vi "ReadReply.vi"(6 "length":i32=-1, 8 "error in (no error)":errorcluster, 9 "Type":enum16{"Header", "Body"}(ring)=enum."Body", 10 "timeout ms (60000)":i32, 11 "TCP in":refnum<k5>) -> (0 "error out":errorcluster, 2 "String":string, 3 "TCP out":refnum<k5>)   [LabVIEW 2019]
panel:
  out "last line":string
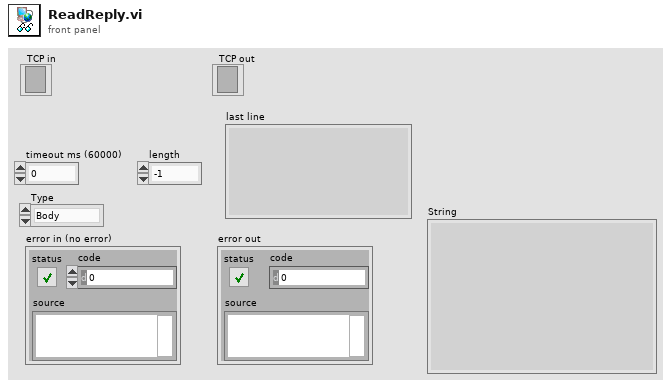
[diagram p1: front panel]
types:
  T1 = enum16{"Standard", "Buffered", "CRLF", "Immediate"}
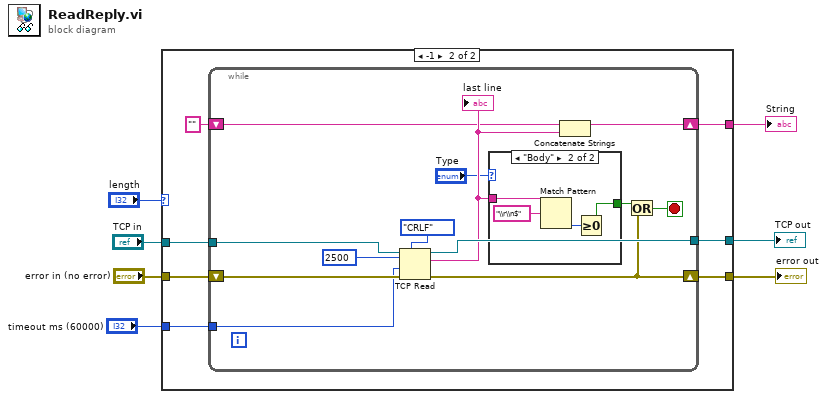
[diagram p0: block diagram]
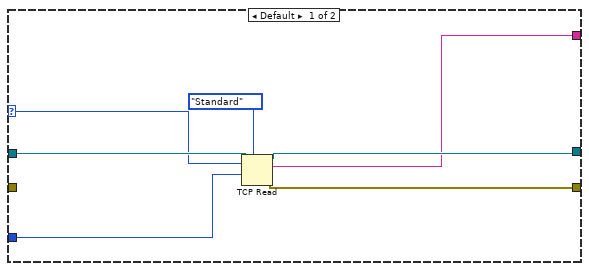
[diagram p2: hidden frame]
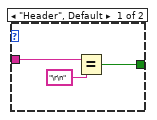
[diagram p3: hidden frame]
diagram:
  n1 = case shown="-1" "length" {
    selector: "length" -> [w11 _]
    tunnel: [w9 w21] -> w7
    tunnel: "error in (no error)" -> [_ w20]
    tunnel: "TCP in" -> [w13 w19]
    tunnel: [w10 w18] -> w4
    tunnel: [w8 w17] -> w3
    tunnel: "timeout ms (60000)" -> [w12 w15]
    frame Default {
      n2 = TCP Read(connection ID=w13, bytes to read=w11, 7:T1."Standard" ("mode (standard)"), 9:w12) -> (connection ID out=w10:refnum<k5>, data out=w8:string, error out=w9:errorcluster)  [unwired: 1 in]
    }
    frame -1 {
      n3 = while {
        shift-right: [w28] -> w21
        shift-left: w20 -> [w34]
        tunnel: w19 -> [w33]
        tunnel: [w32] -> w18
        shift-right: [w31] -> w17
        shift-left: "" ("data out") -> [w26]
        tunnel: w15 -> [w22]
        stop <- w29 stop-if-true
        n4 = TCP Read(connection ID=w33, bytes to read=2500, error in (no error)=w34, 7:T1."CRLF" ("mode (standard)"), 9:w22) -> (connection ID out=w32:refnum<k5>, data out=w27:string, error out=w28:errorcluster)
        "last line" <- w27
        n5 = case shown="\"Body\"" "Type" {
          tunnel: [w36 w38] -> w30
          tunnel: w27 -> [w35 w40]
          frame "Header", Default {
            n6 = Equal?(x=w35, y="\r\n" ("data out")) -> (x = y?=w36:bool)
          }
          frame "Body" {
            n7 = Match Pattern(string=w40, regular expression="\\r\\n$") -> (offset past match=w39:i32)  [unwired: 1 in, 3 out]
            n8 = Greater Or Equal To 0?(x=w39) -> (x >= 0?=w38:bool)
          }
        }
        n9 = Concatenate Strings(w26, w27) -> (w31:string)
        n10 = Or(x=w30, y=w28) -> (x .or. y?=w29:bool)
      }
    }
  }
  "String" <- w3
  "error out" <- w7
  "TCP out" <- w4
